vi "working with objects.vi"() -> ()   [LabVIEW 2016]
uses:
  API/JSON Document Class/json insert/json Insert - String Path.vi
  API/JSON Document Class/json to string/json To Minimized String - string path.vi
  API/JSON Document Class/json member names/json Member Names - string path.vi
  API/JSON Document Class/JSON Document.lvclass
panel:
  out "Member Names":string[](array[string])
  out "json string":string
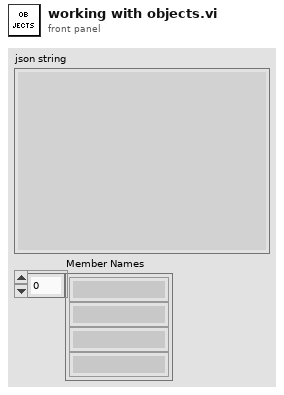
[diagram p1: front panel]
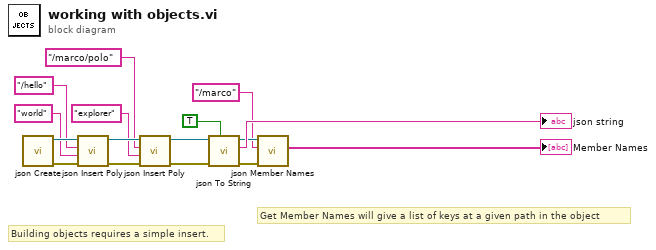
[diagram p0: block diagram]
diagram:
  # "Get Member Names will give a list of keys at a given path in the object"
  # "Building objects requires a simple insert."
  n1 = call "json Create.vi"() -> ("error out"=w13:errorcluster, "JSON Document out"=w16:refnum<class "JSON Document.lvclass">)  [unwired: 10 in]
  n2 = call-poly "json Insert Poly.vi"("error in (no error)"=w13, "anything"="world" ("path"), "path"="/hello", "JSON Document in"=w16) -> ("error out"=w12:errorcluster, "JSON Document out"=w11:refnum<class "JSON Document.lvclass">)  [unwired: 5 in, 1 out]
  n3 = call-poly "json Insert Poly.vi"("error in (no error)"=w12, "anything"="explorer" ("path"), "path"="/marco/polo", "JSON Document in"=w11) -> ("error out"=w7:errorcluster, "JSON Document out"=w8:refnum<class "JSON Document.lvclass">)  [unwired: 5 in, 1 out]
  n4 = call-poly "json To String.vi"("pretty print?"=TRUE, "error in (no error)"=w7, "JSON Document in"=w8) -> ("error out"=w3:errorcluster, "json string"=→"json string":string, "JSON Document out"=w4:refnum<class "JSON Document.lvclass">)  [unwired: 6 in]
  n5 = call-poly "json Member Names.vi"("error in (no error)"=w3, "path"="/marco", "JSON Document in"=w4) -> ("Member Names"=→"Member Names":string[])  [unwired: 6 in, 2 out]
